vi "Close.vi"(8 "error in (no error)":errorcluster, 11 "Controller in":refnum<class "Controller.lvclass">) -> (0 "error out":errorcluster, 3 "Controller out":refnum<class "Controller.lvclass">)   [LabVIEW 2019, in "Controller.lvclass"]
uses:
  Controller.lvclass
  Controller.lvclass/Controller.ctl
  Communication/Communication.lvclass
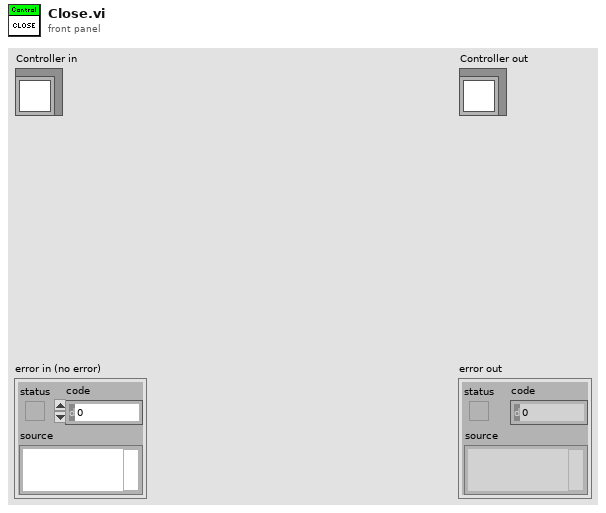
[diagram p1: front panel]
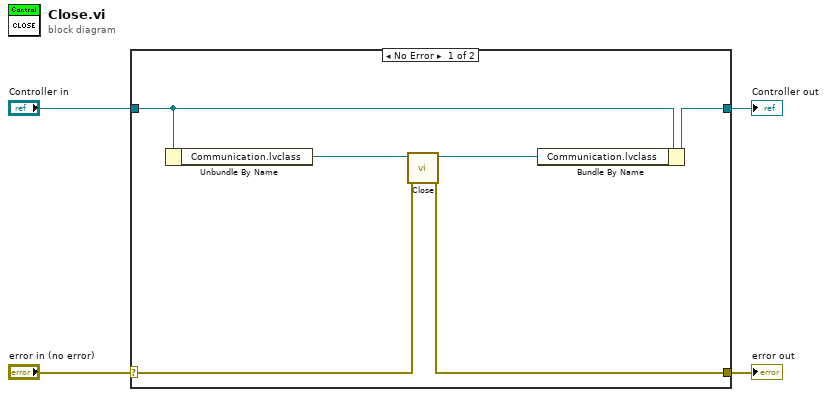
[diagram p0: block diagram]
diagram:
  n1 = case shown="No Error" "error in (no error)" {
    selector: "error in (no error)" -> [w6 w12]
    tunnel: [w5 w12] -> w3
    tunnel: [w10 w11] -> w1
    tunnel: "Controller in" -> [w9 w11]
    frame No Error {
      n2 = Unbundle By Name(w9) -> ("Communication.lvclass"=w8:refnum<class "Communication.lvclass">)
      n3 = call-dynamic "Close.vi"("error in (no error)"=w6, "Communication in"=w8) -> ("error out"=w5:errorcluster, "Communication out"=w7:refnum<class "Communication.lvclass">)  [unwired: 8 in]
      n4 = Bundle By Name(cluster=w9, "Communication.lvclass"=w7) -> (w10:refnum<class "Controller.lvclass">)
    }
    frame Error {
    }
  }
  "error out" <- w3
  "Controller out" <- w1
